vi "CRYPost Processing Curve Name Replace.vi"(7 "Setup in":T1={"No.VI"=0, "Category"="", "StepName"="", "Seq setup flattened"="", "Comment"="", "Steps config."=[], "Jump config"=[], "Start"=0.0, "Increment"=0.0, "Name"="Pa", "Unit"="Pa", "Y data"=1, "Y prefix"="", "Y dB ref"=1.0, "Y unit"="", "Repeat State Array"=[]} {"Repeat State Array"."Start" format="%#_5g"; "Y dB ref" format="%.1f"; "Y data" items=["dB", "Lin"]; "Start" format="%#_5g"}, 8 "Hardware in":string, 9 "Step Setup in":string, 11 "Type In":string) -> (3 "Inserted Names Out":string[](array[string]))   [LabVIEW 2013]
uses:
  Typedef Control/CRYStep.ctl
  Typedef Control/CRYData Cluster Array.ctl
  Typedef Control/CRYData Cluster.ctl
  Typedef Control/CRYWaveform Cluster Array.ctl
  Typedef Control/CRYWaveform Cluster.ctl
  Typedef Control/CRYResult Cluster Array.ctl
  Typedef Control/CRYResult Cluster.ctl
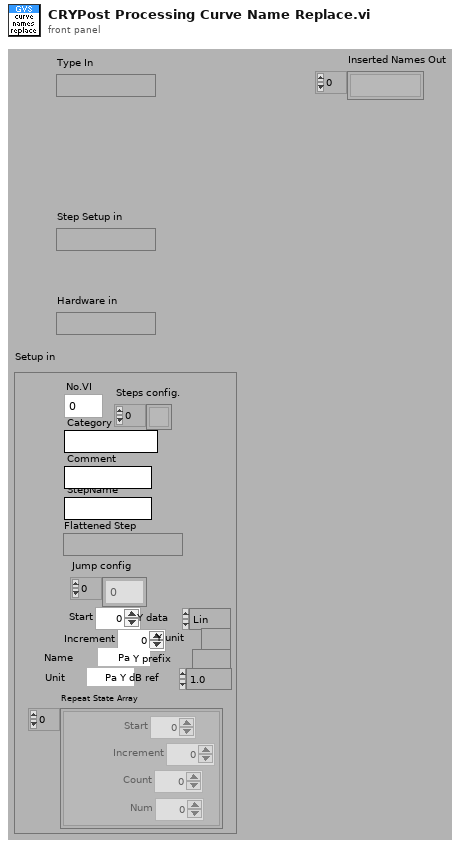
[diagram p1: front panel]
types:
  T1 = typedef "CRYStep.ctl" = cluster{"No.VI":i32, "Category":string, "StepName":string, "Seq setup flattened":string, "Comment":string, "Steps config.":bool[], "Jump config":i32[], "Start":dbl, "Increment":dbl, "Name":string, "Unit":string, "Y data":u16, "Y prefix":string, "Y dB ref":dbl, "Y unit":string, "Repeat State Array":cluster{"Start":dbl, "Increment":dbl, "Count":i32, "Num":i32}[]}
  T2 = typedef "CRYResult Cluster Array.ctl" = T3[]
  T3 = typedef "CRYResult Cluster.ctl" = cluster{"Name":string, "Margin":dbl, "unit":string, "Verdict":bool, "Limit":string, "Max/Min":string, "protected":bool, "Step No.":i32, "Test Info":string, "AutoProtect":bool}
  T4 = typedef "CRYWaveform Cluster Array.ctl" = T5[]
  T5 = typedef "CRYWaveform Cluster.ctl" = cluster{"Waveform":cluster{"X0":dbl, "dX":dbl, "Y":sgl[]}, "X data":u16, "Y data":u16, "Y axis":u16, "X unit":string, "Y unit":string, "Y dB ref":dbl, "display Y":bool, "display X":bool, "Overload?":bool, "Test Info":string, "Step No.":i32, "Name":string, "protected":bool, "Sqc history":string[], "Signal Channel ID":i32, "Plot Settings":cluster{"Color":u32, "Interpolation":u8, "Point Style":u8, "Line Style":u8, "Point Color":u32, "Line Width":u8, "Bar Plot Style":u8, "Fill To":i16}, "AutoProtect":bool}
  T6 = typedef "CRYData Cluster Array.ctl" = T7[]
  T7 = typedef "CRYData Cluster.ctl" = cluster{"Name":string, "Curve":cluster{"x":dbl, "y":dbl, "z":dbl}[], "X data":u16, "Y data":u16, "Z data":u16, "X axis":u16, "Y axis":u16, "Z axis":u16, "X unit":string, "Y unit":string, "Z unit":string, "X dB ref":dbl, "Y dB ref":dbl, "Z dB ref":dbl, "single val":bool, "protected":bool, "display X":bool, "display Y":bool, "display Z":bool, "Test Info":string, "Step No.":i32, "Plot Settings":cluster{"Color":u32, "Interpolation":u8, "Point Style":u8, "Line Style":u8, "Point Color":u32, "Line Width":u8, "Bar Plot Style":u8, "Fill To":i16}, "AutoProtect":bool}
  T8 = cluster{"Start":dbl, "Increment":dbl, "Count":i32, "Num":i32}[]
  T9 = typedef "CRYPost Processing Cluster.ctl" = cluster{"Name":string, "Op Type":u16, "Curve A":string, "Curve B":string, "Axis Mode":u16, "Work Mode":u16, "Width":u16, "Weighting win":u16, "Search Mode":u16, "Freq Mode":u16, "New Sampling Rate":dbl, "Use Default Name":bool, "x":bool, "y":bool, "z":bool, "All points":bool, "A_single val axis":u16, "B_single val axis":u16, "Use Default Value":bool, "Result Name":string, "Smoothing Width":i32, "Window":u16, "Para_dB":sgl, "Para_%":sgl, "Exponent":sgl, "Hz":dbl, "Direct Weighting":bool, "Auto Inc":bool, "Inc(deg)":i32, "Total Rotation":i32, "Ref Freq Mode":u16, "Ref Waveform":string, "Sampling Rate":dbl, "Weighting Curve":string, "Ref Freq":dbl, "Curve Group":string[], "Search Items":string[], "Custom unit info":cluster{"use custom":bool, "lin/log":u16, "unit":string, "dB ref":dbl, "common dB":u16}, "Unit":string, "Type A":enum16{"Curves", "Values", "Results", "WFM"}, "Type B":enum16{"Curves", "Values", "Results", "WFM"}, "Unary Operator":u16, "Binary Operator":u16, "Statistical Operator":u16, "Constant ":dbl, "New Resolution":u16, "user equation cluster":T10, "Help":string, "Tab Value":enum32{"Setting", "Help"}, "Zwciker_X-axis":u16, "Zwicker_spectrum":bool, "Freq Sampling Mode":u16, "Freq Sampling Rate":dbl, "Smoothing":bool, "Work in Statics":u16, "Result Data":string[]}
  T10 = typedef "CRYUser Equation Cluster.ctl" = cluster{"Custom unit input array":cluster{"use custom":bool, "lin/log":u16, "unit":string, "dB ref":dbl, "common dB":u16}[], "Custom unit results array ":cluster{"use custom":bool, "lin/log":u16, "unit":string, "dB ref":dbl, "common dB":u16}[], "Desired Result Variables":string[], "Desired Result Names":string[], "Input Curve Names":string[], "Input Curve Variables":string[], "equation":string, "Input axis":u16[], "Results axis":u16[], "# input curves":i32, "# Desired result curves ":i32, "Input Values":string[], "Result Values":string[]}
  T11 = cluster{"Res Name":string, "Type out":enum16{"Curves", "Values", "Results", "WFM"}}[]
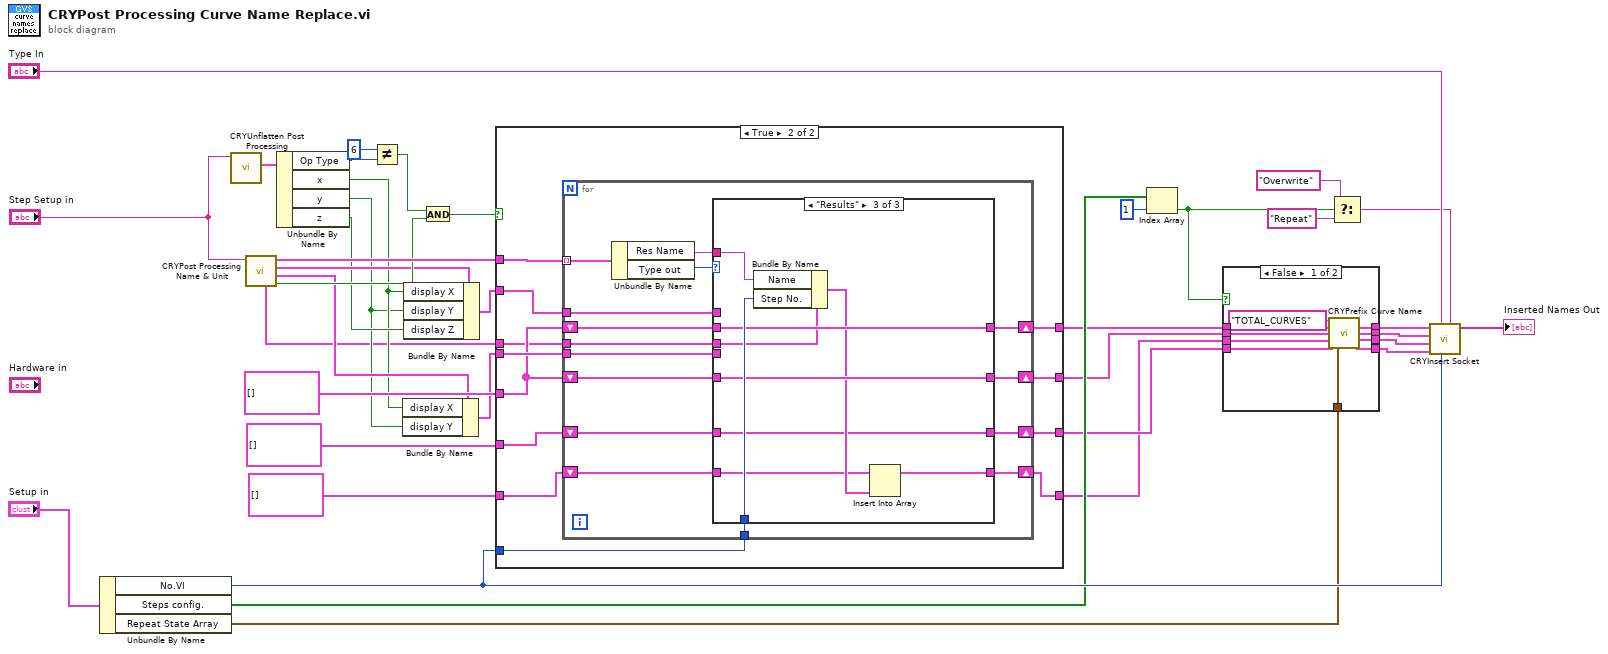
[diagram p0: block diagram]
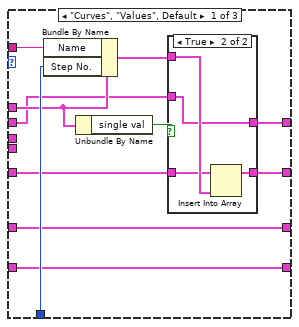
[diagram p4: hidden frame]
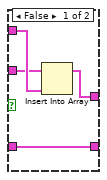
[diagram p5: hidden frame]
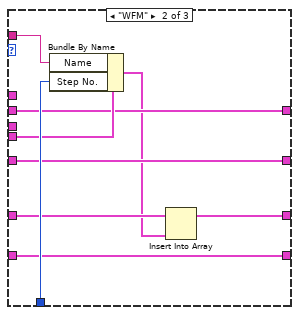
[diagram p6: hidden frame]
diagram:
  n1 = Unbundle By Name("Setup in") -> ("No.VI"=w14:i32, "Steps config."=w13:bool[], "Repeat State Array"=w5:T8)
  n2 = call "CRYUnflatten Post Processing.vi"("Unflatten Post Processing"="Step Setup in") -> ("Post-Processing"=w38:T9)  [unwired: 8 in, 2 out]
  n3 = call "CRYPost Processing Name & Unit.vi"("Step setup"="Step Setup in") -> ("Run abble?"=w32:bool, "Waveform"=w19:T5, "Data"=w22:T7, "Result name and type"=w34:T11, "Result"=w1:T3)  [unwired: 6 in]
  n4 = Unbundle By Name(w38) -> ("Op Type"=w37:u16, "x"=w17:bool, "y"=w16:bool, "z"=w20:bool)
  n5 = Not Equal?(x=u16 6, y=w37) -> (x != y?=w33:bool)
  n6 = Bundle By Name(cluster=w19, "display X"=w17, "display Y"=w16) -> (w18:T5)
  n7 = Bundle By Name(cluster=w22, "display X"=w17, "display Y"=w16, "display Z"=w20) -> (w21:T7)
  n8 = And(x=w33, y=w32) -> (x .and. y?=w31:bool)
  n9 = case shown="True" w31 {
    tunnel: w14 -> [_ w53]
    tunnel: [w41 w52] -> w12
    tunnel: [w41 w51] -> w11
    tunnel: [w40 w50] -> w10
    tunnel: w34 -> [_ w49]
    tunnel: w21 -> [_ w48]
    tunnel: w18 -> [_ w47]
    tunnel: T6 [] ("Data array") -> [w41 w46]
    tunnel: T4 [] ("Waveform Array") -> [w40 w45]
    tunnel: T2 [] ("Results") -> [w39 w44]
    tunnel: [w39 w42] -> w3
    tunnel: w1 -> [_ w43]
    frame False {
    }
    frame True {
      n10 = for {
        tunnel: w49 -> [w68] mode=indexing
        tunnel: w53 -> [w66]
        tunnel: w47 -> [w65]
        tunnel: w48 -> [w64]
        shift-right: [w62] -> w50
        shift-left: w45 -> [w61]
        shift-right: [w59] -> w52
        shift-left: w46 -> [w60]
        shift-right: [w57] -> w51
        shift-left: w46 -> [w58]
        shift-right: [w55] -> w42
        shift-left: w44 -> [w56]
        tunnel: w43 -> [w54]
        n11 = Unbundle By Name(w68) -> ("Res Name"=w67:string, "Type out"=w63:enum16{"Curves", "Values", "Results", "WFM"})
        n12 = case shown="\"Results\"" w63 {
          tunnel: w67 -> [w79 w96 w105]
          tunnel: w66 -> [w78 w95 w104]
          tunnel: w65 -> [_ w94 _]
          tunnel: w64 -> [w77 _ _]
          tunnel: [w75 w92 w98] -> w62
          tunnel: w61 -> [w75 w93 w98]
          tunnel: w60 -> [w74 w91 w103]
          tunnel: [w73 w91 w103] -> w59
          tunnel: w58 -> [w72 w90 w102]
          tunnel: [w71 w90 w102] -> w57
          tunnel: w56 -> [w69 w88 w100]
          tunnel: [w69 w88 w99] -> w55
          tunnel: w54 -> [_ _ w97]
          frame "Curves", "Values", Default {
            n13 = Bundle By Name(cluster=w77, "Name"=w79, "Step No."=w78) -> (w70:T7)
            n14 = Unbundle By Name(w77) -> ("single val"=w76:bool)
            n15 = case shown="True" w76 {
              tunnel: w70 -> [w83 w87]
              tunnel: w74 -> [w82 w84]
              tunnel: [w81 w84] -> w73
              tunnel: w72 -> [w80 w86]
              tunnel: [w80 w85] -> w71
              frame False {
                n16 = Insert Into Array(array=w82, new element=w83) -> (w81:T6)  [unwired: 1 in]
              }
              frame True {
                n17 = Insert Into Array(array=w86, new element=w87) -> (w85:T6)  [unwired: 1 in]
              }
            }
          }
          frame "WFM" {
            n18 = Bundle By Name(cluster=w94, "Name"=w96, "Step No."=w95) -> (w89:T5)
            n19 = Insert Into Array(array=w93, new element=w89) -> (w92:T4)  [unwired: 1 in]
          }
          frame "Results" {
            n20 = Bundle By Name(cluster=w97, "Name"=w105, "Step No."=w104) -> (w101:T3)
            n21 = Insert Into Array(array=w100, new element=w101) -> (w99:T2)  [unwired: 1 in]
          }
        }
      }
    }
  }
  n22 = Index Array(array=w13, index=1) -> (element=w6:bool)
  n23 = case shown="False" w6 {
    tunnel: w12 -> [w114 w119]
    tunnel: w11 -> [w113 w118]
    tunnel: w10 -> [w112 w117]
    tunnel: [w111 w119] -> w9
    tunnel: [w110 w118] -> w8
    tunnel: [w109 w117] -> w7
    tunnel: w5 -> [w108 _]
    tunnel: w3 -> [w107 w116]
    tunnel: [w106 w116] -> w2
    frame False {
      n24 = call "CRYPrefix Curve Name.vi"("Type In"="TOTAL_CURVES", "Curves In"=w114, "Values In"=w113, "Results In"=w107, "Waves In"=w112, "Repeat State Array In"=w108) -> ("Curves Out"=w111:T6, "Values Out"=w110:T6, "Results Out"=w106:T2, "Waves Out"=w109:T4)  [unwired: 6 in]
    }
    frame True {
    }
  }
  n25 = Select(t="Overwrite" ("Y unit"), s=w6, f="Repeat") -> (s? t:f=w24:string)
  n26 = call "CRYInsert Socket.vi"("sOption2"=w24, "Step No."=w14, "sOption1"="Type In", "Waves"=w7, "Results"=w2, "Values"=w8, "Curves"=w9) -> ("Inserted Names Out"=→"Inserted Names Out":string[])  [unwired: 4 in]
